vi "trigger-test.vi"() -> ()   [LabVIEW 2020, in "VDTD.lvlib"]
uses:
  VDTD.lvlib
panel:
  in  "to trigger":bool
  out "trigger":bool
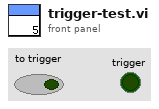
[diagram p1: front panel]
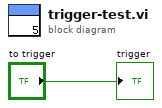
[diagram p0: block diagram]
diagram:
  "trigger" <- "to trigger"
